vi "Set to Factory Default.vi"(6 "VestaTemperature Fixed":T1={"Water Heater Temp (°F)"=125, "Differential  (°F)"=25.0} {"Water Heater Temp (°F)" min=32 max=203}, 8 "error in (no error)":errorcluster, 9 "Send_Vesta_Message":u8, 10 "Vesta in":refnum<queue>, 11 "Data Cluster In":T2 {"VestaTemperature"."Water Heater Temp (°F)" min=32 max=203}) -> (0 "error out":errorcluster, 3 "Data Cluster Out":T2 {"VestaTemperature"."Water Heater Temp (°F)" min=32 max=203})   [LabVIEW 2023]
uses:
  controls/UI Data.ctl
  Drivers/Resideo Gas Valve/Type Definitions/Vesta Info.ctl
  Drivers/Resideo Gas Valve/Type Definitions/Temperature Control.ctl
  controls/Timer Application Cluster.ctl
  controls/Burner Duty Cycle.ctl
  Hybrid Water Heater/Type Definitions/HEWH MW100 Data Cluster.ctl
  Hybrid Water Heater/Custom Instrument Control/MW100/Type Definitions/HEWH Module 4 Relay Status.ctl
  Message Queue/Message Cluster.ctl
  Message Queue/Enqueue Message (Single).vi
  Message Queue/Message Queue.lvlib
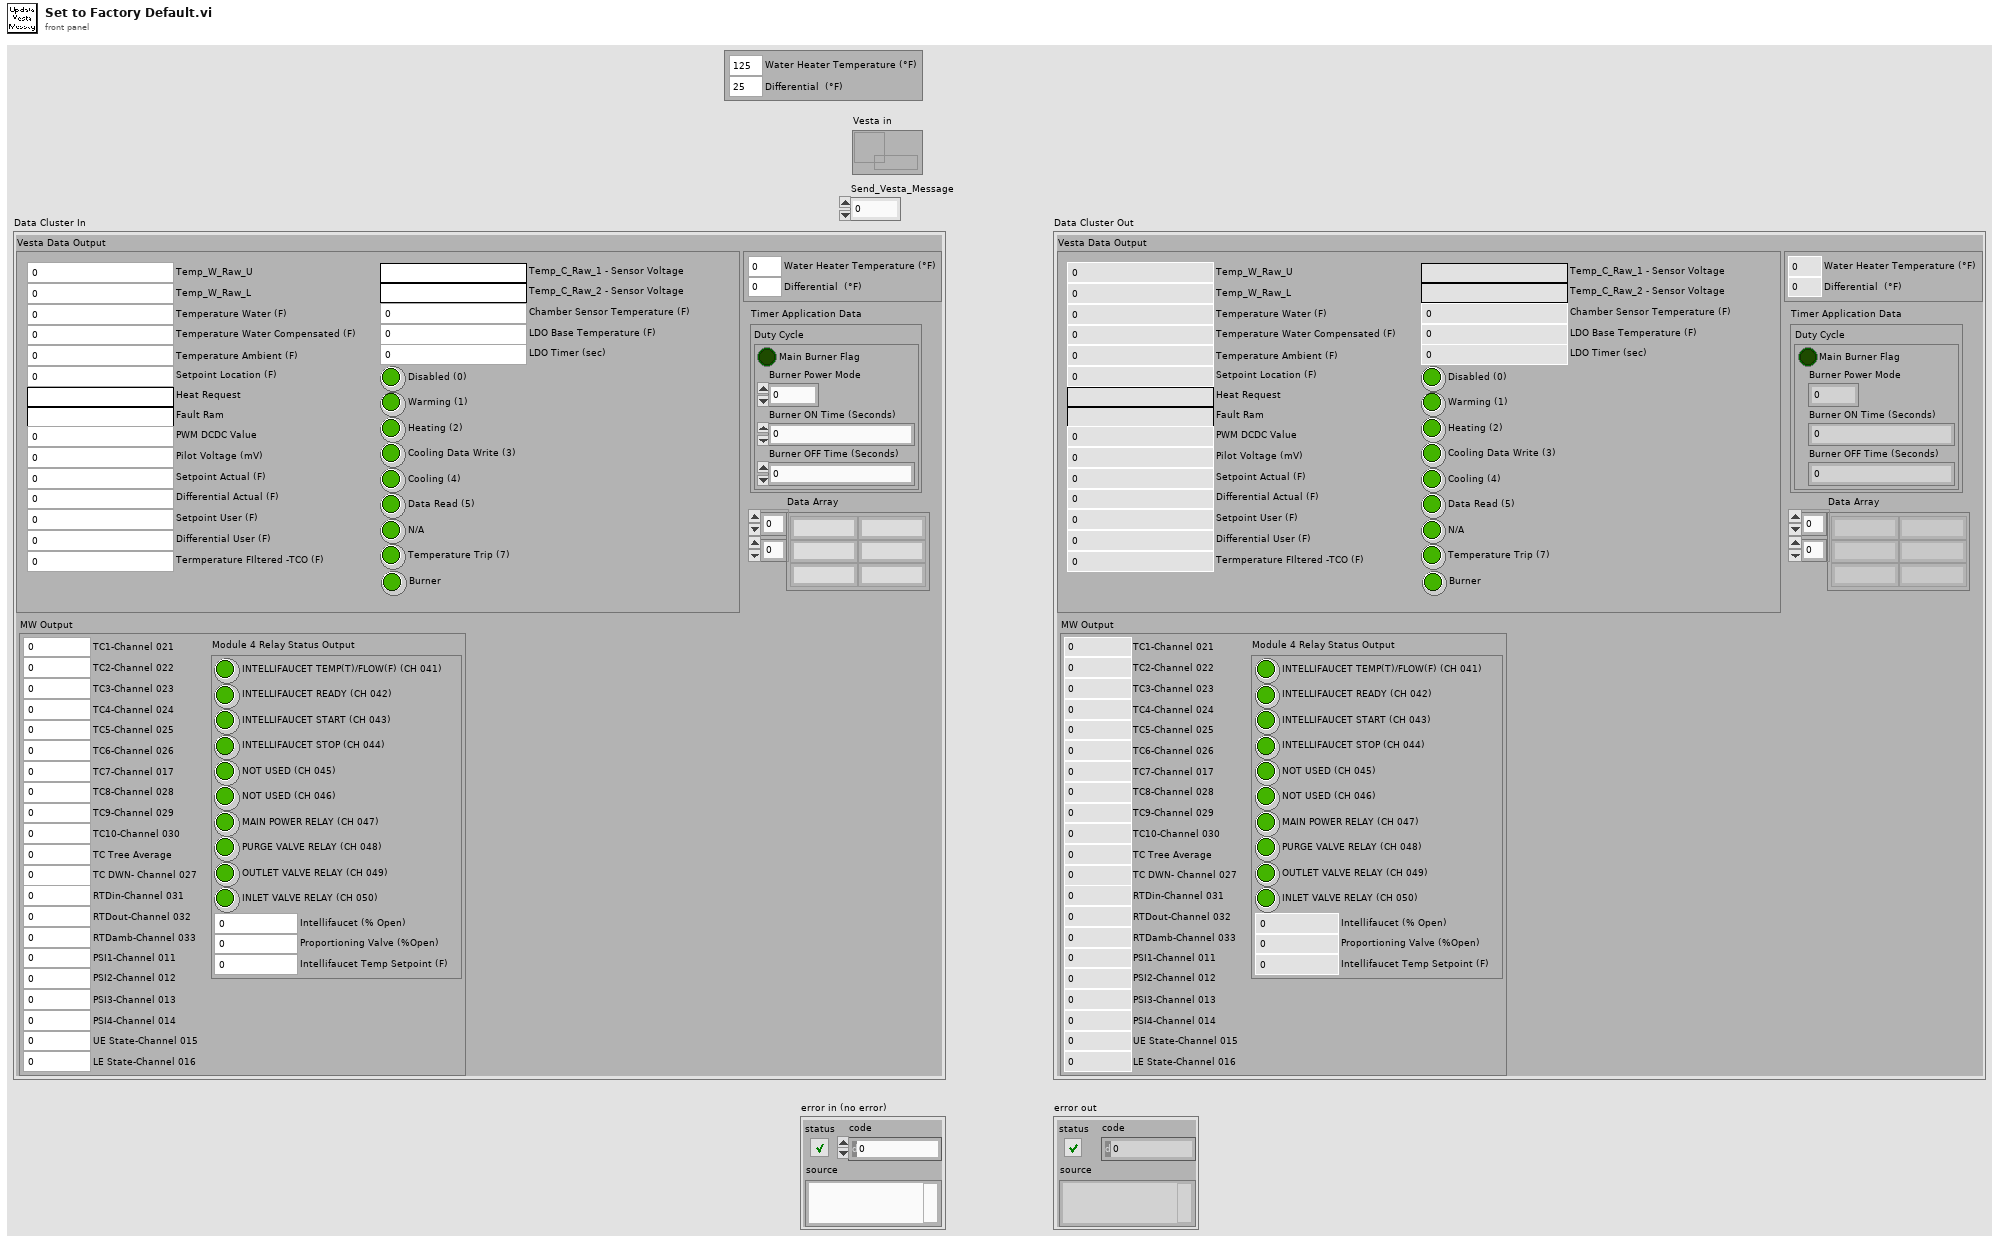
[diagram p1: front panel]
types:
  T1 = typedef "Temperature Control.ctl" = cluster{"Water Heater Temp (°F)":u16, "Differential  (°F)":dbl}
  T2 = typedef "UI Data.ctl" = cluster{"Vesta Data Output":T3, "VestaTemperature":T1, "Timer Application Data":T4, "Data Array":string[][], "MW Output":T6}
  T3 = typedef "Vesta Info.ctl" = cluster{"Temp_W_Raw_U":u16, "Temp_W_Raw_L":u16, "Temperature Water (F)":dbl, "Temperature Water Compensated (F)":dbl, "Temperature Ambient (F)":dbl, "Setpoint Location (F)":dbl, "Heat Request":string, "Fault Ram":string, "PWM DCDC Value":u16, "Pilot Voltage (mV)":dbl, "Setpoint Actual (F)":dbl, "Differential Actual (F)":dbl, "Setpoint User (F)":dbl, "Differential User (F)":dbl, "Termperature FIltered -TCO (F)":dbl, "Temp_C_Raw_1 - Sensor Voltage":string, "Temp_C_Raw_2 - Sensor Voltage":string, "Chamber Sensor Temperature (F)":dbl, "LDO Base Temperature (F)":dbl, "LDO Timer (sec)":i16, "Disabled (0)":bool, "Warming (1)":bool, "Heating (2)":bool, "Cooling Data Write (3)":bool, "Cooling (4)":bool, "Data Read (5)":bool, "N/A":bool, "Temperature Trip (7)":bool, "Burner":bool}
  T4 = typedef "Timer Application Cluster.ctl" = cluster{"Duty Cycle":T5}
  T5 = typedef "Burner Duty Cycle.ctl" = cluster{"Burner ON Time (Seconds)":dbl, "Burner OFF Time (Seconds)":dbl, "Main Burner Flag":bool, "Burner Power Mode":u8}
  T6 = typedef "HEWH MW100 Data Cluster.ctl" = cluster{"TC1-Channel 021":dbl, "TC2-Channel 022":dbl, "TC3-Channel 023":dbl, "TC4-Channel 024":dbl, "TC5-Channel 025":dbl, "TC6-Channel 026":dbl, "TC7-Channel 017":dbl, "TC8-Channel 028":dbl, "TC9-Channel 029":dbl, "TC10-Channel 030":dbl, "TC Tree Average":dbl, "TC DWN- Channel 027":dbl, "RTDin-Channel 031":dbl, "RTDout-Channel 032":dbl, "RTDamb-Channel 033":dbl, "PSI1-Channel 011":dbl, "PSI2-Channel 012":dbl, "PSI3-Channel 013":dbl, "PSI4-Channel 014":dbl, "UE State-Channel 015":dbl, "LE State-Channel 016":dbl, "Module 4 Relay Status Output":T7}
  T7 = typedef "HEWH Module 4 Relay Status.ctl" = cluster{"INTELLIFAUCET TEMP(T)/FLOW(F) (CH 041)":bool, "INTELLIFAUCET READY (CH 042)":bool, "INTELLIFAUCET START (CH 043)":bool, "INTELLIFAUCET STOP (CH 044)":bool, "MAIN POWER RELAY (CH 047)":bool, "NOT USED (CH 045)":bool, "NOT USED (CH 046)":bool, "PURGE VALVE RELAY (CH 048)":bool, "OUTLET VALVE RELAY (CH 049)":bool, "INLET VALVE RELAY (CH 050)":bool, "Intellifaucet (% Open)":dbl, "Proportioning Valve (%Open)":dbl, "Intellifaucet Temp Setpoint (F)":dbl}
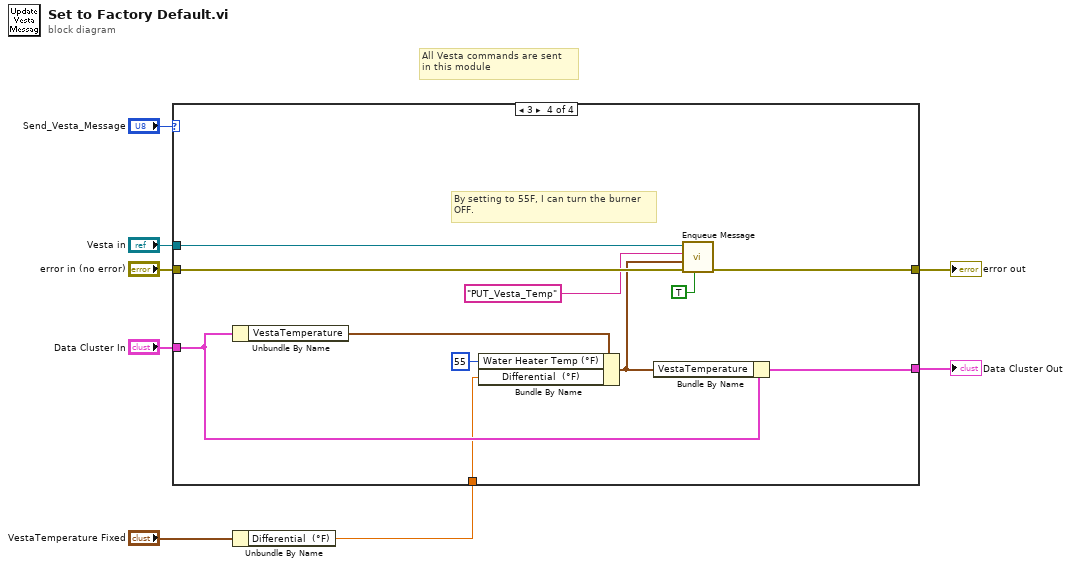
[diagram p0: block diagram]
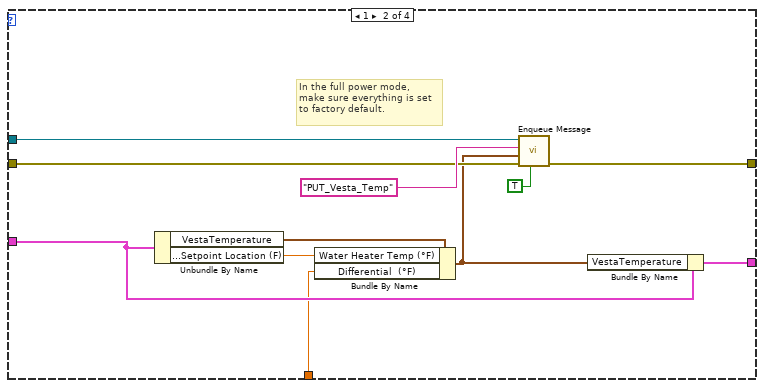
[diagram p3: hidden frame]
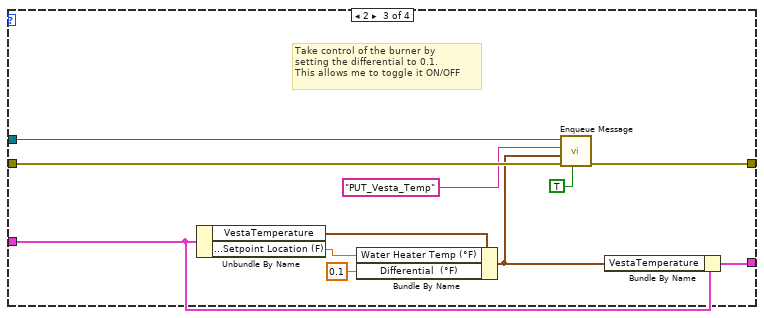
[diagram p4: hidden frame]
diagram:
  # "All Vesta commands are sent \nin this module"
  n1 = Unbundle By Name("VestaTemperature Fixed") -> ("Differential  (°F)"=w1:dbl)
  n2 = case shown="3" "Send_Vesta_Message" {
    tunnel: "Vesta in" -> [_ w19 w32 w43]
    tunnel: "error in (no error)" -> [w10 w18 w31 w42]
    tunnel: [w10 w17 w30 w41] -> w7
    tunnel: "Data Cluster In" -> [w9 w14 w22 w39]
    tunnel: [w9 w12 w29 w40] -> w3
    tunnel: w1 -> [_ w11 _ w33]
    frame 0, Default {
      # "Do nothing. All is good."
    }
    frame 1 {
      # "In the full power mode,\nmake sure everything is set\nto factory default."
      n3 = Unbundle By Name(w14) -> ("VestaTemperature"=w15:T1, "Vesta Data Output.Setpoint Location (F)"=w16:dbl)
      n4 = Bundle By Name(cluster=w15, "Water Heater Temp (°F)"=w16, "Differential  (°F)"=w11) -> (w13:T1)
      n5 = call-poly "Enqueue Message.vi"("Priority Message? (F)"=TRUE, "error in (no error)"=w18, "Message Data"=w13, "Message"="PUT_Vesta_Temp", "Message Queue"=w19) -> ("error out"=w17:errorcluster)  [unwired: 5 in, 1 out]
      n6 = Bundle By Name(cluster=w14, "VestaTemperature"=w13) -> (w12:T2)
    }
    frame 2 {
      # "Take control of the burner by \nsetting the differential to 0.1.\nThis allows me to toggle it ON/OFF"
      n7 = Unbundle By Name(w22) -> ("VestaTemperature"=w24:T1, "Vesta Data Output.Setpoint Location (F)"=w25:dbl)
      n8 = Bundle By Name(cluster=w24, "Water Heater Temp (°F)"=w25, "Differential  (°F)"=0.1) -> (w23:T1)
      n9 = call-poly "Enqueue Message.vi"("Priority Message? (F)"=TRUE, "error in (no error)"=w31, "Message Data"=w23, "Message"="PUT_Vesta_Temp", "Message Queue"=w32) -> ("error out"=w30:errorcluster)  [unwired: 5 in, 1 out]
      n10 = Bundle By Name(cluster=w22, "VestaTemperature"=w23) -> (w29:T2)
    }
    frame 3 {
      # "By setting to 55F, I can turn the burner\nOFF."
      n11 = Unbundle By Name(w39) -> ("VestaTemperature"=w35:T1)
      n12 = Bundle By Name(cluster=w35, "Water Heater Temp (°F)"=u16 55, "Differential  (°F)"=w33) -> (w34:T1)
      n13 = Bundle By Name(cluster=w39, "VestaTemperature"=w34) -> (w40:T2)
      n14 = call-poly "Enqueue Message.vi"("Priority Message? (F)"=TRUE, "error in (no error)"=w42, "Message Data"=w34, "Message"="PUT_Vesta_Temp", "Message Queue"=w43) -> ("error out"=w41:errorcluster)  [unwired: 5 in, 1 out]
    }
  }
  "error out" <- w7
  "Data Cluster Out" <- w3
